vi "SignalOutput.vi"(1 "signal cluster":T1, 2 "Gain Type":string, 3 "SetIntr Cluster":cluster{dbl, dbl, dbl, dbl, dbl, dbl, dbl}) -> (0 "Signal output":dbl)   [LabVIEW 2011]
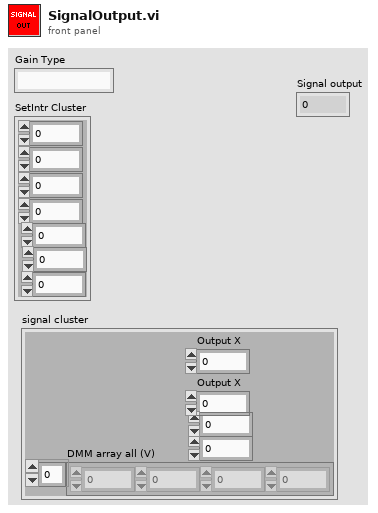
[diagram p1: front panel]
types:
  T1 = cluster{"Output X":dbl, "Output X":dbl, dbl, dbl, "DMM array all (V)":dbl[]}
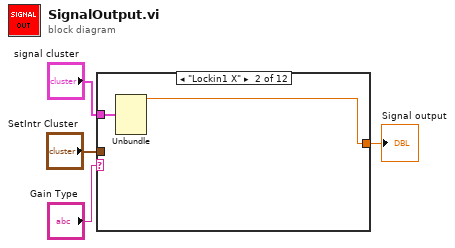
[diagram p0: block diagram]
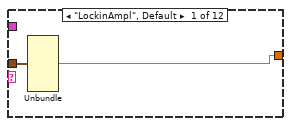
[diagram p2: hidden frame]
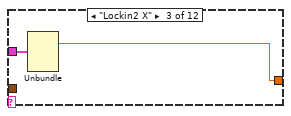
[diagram p3: hidden frame]
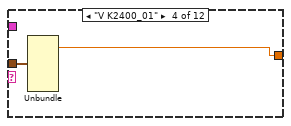
[diagram p4: hidden frame]
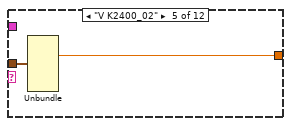
[diagram p5: hidden frame]
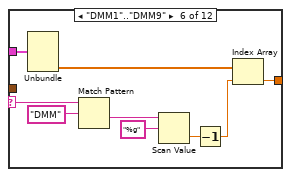
[diagram p6: hidden frame]
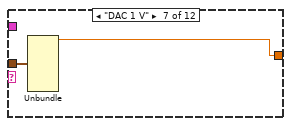
[diagram p7: hidden frame]
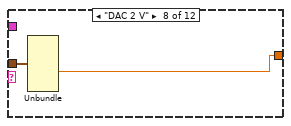
[diagram p8: hidden frame]
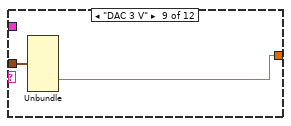
[diagram p9: hidden frame]
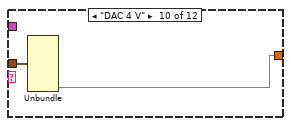
[diagram p10: hidden frame]
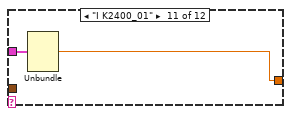
[diagram p11: hidden frame]
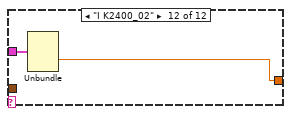
[diagram p12: hidden frame]
diagram:
  n1 = case shown="\"Lockin1 X\"" "Gain Type" {
    selector: "Gain Type" -> [_ _ _ _ _ w19 _ _ _ _ _ _]
    tunnel: "SetIntr Cluster" -> [w6 _ _ w12 w14 _ w25 w27 w29 w31 _ _]
    tunnel: "signal cluster" -> [_ w8 w10 _ _ w23 _ _ _ _ w33 w35]
    tunnel: [w5 w7 w9 w11 w13 w16 w24 w26 w28 w30 w32 w34] -> w1
    frame "LockinAmpl", Default {
      n2 = Unbundle(w6) -> (w5:dbl)  [unwired: 6 out]
    }
    frame "Lockin1 X" {
      n3 = Unbundle(w8) -> ("Output X"=w7:dbl)  [unwired: 4 out]
    }
    frame "Lockin2 X" {
      n4 = Unbundle(w10) -> ("Output X"=w9:dbl)  [unwired: 4 out]
    }
    frame "V K2400_01" {
      n5 = Unbundle(w12) -> (w11:dbl)  [unwired: 6 out]
    }
    frame "V K2400_02" {
      n6 = Unbundle(w14) -> (w13:dbl)  [unwired: 6 out]
    }
    frame "DMM1".."DMM9" {
      n7 = Unbundle(w23) -> ("DMM array all (V)"=w18:dbl[])  [unwired: 4 out]
      n8 = Match Pattern(string=w19, regular expression="DMM") -> (after substring=w21:string)  [unwired: 1 in, 3 out]
      n9 = Scan Value(string=w21, format string="%g") -> (value=w17:dbl)  [unwired: 1 in, 1 out]
      n10 = Decrement(x=w17) -> (x-1=w15:dbl)
      n11 = Index Array(array=w18, index=w15) -> (element=w16:dbl)
    }
    frame "DAC 1 V" {
      n12 = Unbundle(w25) -> (w24:dbl)  [unwired: 6 out]
    }
    frame "DAC 2 V" {
      n13 = Unbundle(w27) -> (w26:dbl)  [unwired: 6 out]
    }
    frame "DAC 3 V" {
      n14 = Unbundle(w29) -> (w28:dbl)  [unwired: 6 out]
    }
    frame "DAC 4 V" {
      n15 = Unbundle(w31) -> (w30:dbl)  [unwired: 6 out]
    }
    frame "I K2400_01" {
      n16 = Unbundle(w33) -> (w32:dbl)  [unwired: 4 out]
    }
    frame "I K2400_02" {
      n17 = Unbundle(w35) -> (w34:dbl)  [unwired: 4 out]
    }
  }
  "Signal output" <- w1
